vi "Created.vi"(8 "Created Alias":string, 9 "Priority?":bool, 10 "Msg Strategy":refnum<class "Msg Strategy.lvclass">, 11 "Base jettl in":refnum<class "Base jettl.lvclass">) -> (3 "Base jettl out":refnum<class "Base jettl.lvclass">)   [LabVIEW 2021, in "jettl.lvlib" / "Base jettl.lvclass"]
uses:
  Base jettl.lvclass
  Msg Strategy/Msg Strategy.lvclass
  Base jettl.lvclass/Base jettl.ctl
  Addresses Strategy/Addresses Strategy/Addresses Strategy.lvclass
  Error/Error.lvlib
  Sender/Sender.lvlib
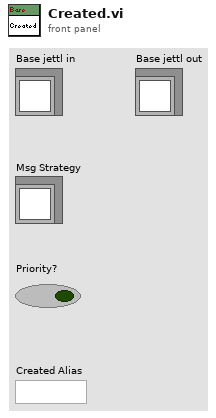
[diagram p1: front panel]
types:
  T1 = typedef "jettl.lvlib/Addresses Strategy.lvlib/Created.ctl" = map{string, refnum<user-event>}
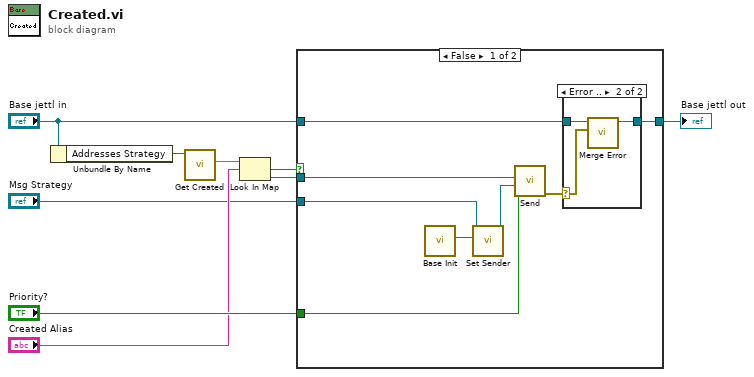
[diagram p0: block diagram]
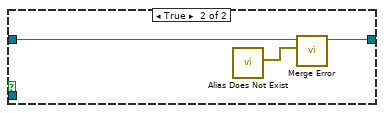
[diagram p3: hidden frame]
diagram:
  n1 = Unbundle By Name("Base jettl in") -> ("Addresses Strategy"=w7:refnum<class "Addresses Strategy.lvclass">)
  n2 = call-dynamic "Get Created.vi"("Addresses Strategy in"=w7) -> ("Created"=w5:T1)  [unwired: 10 in]
  n3 = Look In Map(map=w5, key="Created Alias") -> (key not found?=w2:bool, value=w4:refnum<user-event>)  [unwired: 1 in]
  n4 = case shown="False" w2 {
    tunnel: "Base jettl in" -> [w16 w24]
    tunnel: [w15 w23] -> w8
    tunnel: "Msg Strategy" -> [w12 _]
    tunnel: "Priority?" -> [w14 _]
    tunnel: w4 -> [w13 _]
    frame False {
      n5 = call "Base Init.vi"() -> ("Sender"=w10:refnum<class "Sender.lvclass">)  [unwired: 11 in]
      n6 = call-dynamic "Set Sender.vi"("Sender"=w10, "Msg Strategy in"=w12) -> ("Msg Strategy out"=w11:refnum<class "Msg Strategy.lvclass">)  [unwired: 9 in]
      n7 = call "Send.vi"("Priority?"=w14, "Msg Strategy"=w11, "Msg Event"=w13) -> ("error out"=w17:errorcluster)  [unwired: 8 in]
      n8 = case shown="Error .." w17 {
        selector: w17 -> [_ w19]
        tunnel: [w18 w21] -> w15
        tunnel: w16 -> [w18 w20]
        frame No Error {
        }
        frame Error {
          n9 = call-dynamic "Merge Error.vi"("Error"=w19, "Base jettl in"=w20) -> ("Base jettl out"=w21:refnum<class "Base jettl.lvclass">)  [unwired: 9 in]
        }
      }
    }
    frame True {
      n10 = call "Alias Does Not Exist.vi"() -> ("Error"=w22:errorcluster)  [unwired: 11 in]
      n11 = call-dynamic "Merge Error.vi"("Error"=w22, "Base jettl in"=w24) -> ("Base jettl out"=w23:refnum<class "Base jettl.lvclass">)  [unwired: 9 in]
    }
  }
  "Base jettl out" <- w8
